vi "ArdnoTimedValves.vi"() -> ()   [LabVIEW 2018, in "Arduino.lvlib"]
uses:
  Backup LabVIEW Arduino Connection/LINX/Public/Peripherals/Digital/Digital Write N Chans.vi
  Arduino.lvlib
  Backup LabVIEW Arduino Connection/LINX/LVH-LINX.lvlib
panel:
  in  "Period [ms]":u32
  out "Error Out":errorcluster
  out "Device Name":string
  in  "error in (no error)":errorcluster
  in  "VISA resource name":refnum<visa-resource-name>
  in  "Manually controlled Valves":u8[](array[numeric])
  out "Open?":bool
  in  "Manual Open":bool
  in  "stop":bool
  # "ALWAYS TERMINATE THE\nPROGRAM WITH THIS STOP BUTTON!"
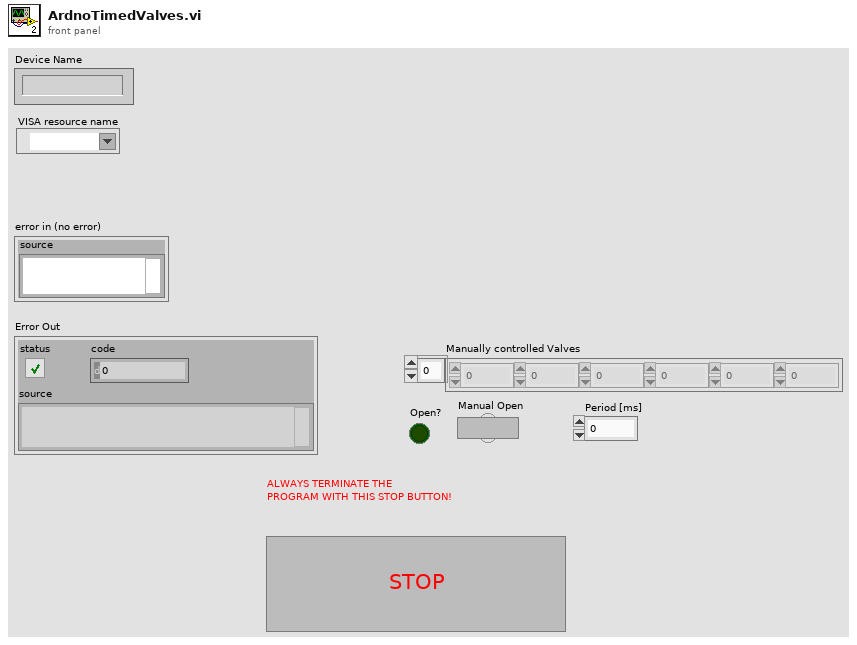
[diagram p1: front panel]
types:
  T1 = typedef "LVH-LINX.lvlib/LINX Ref.ctl" = cluster{"Platform":T2, "Interface":T3, "LINX Device Config":T4}
  T2 = typedef "LVH-LINX.lvlib/Platform.ctl" = enum16{"LINX", "myRIO"}
  T3 = typedef "LVH-LINX.lvlib/Interface.ctl" = enum16{"Serial", "TCP"}
  T4 = typedef "LVH-LINX.lvlib/Device.lvlib/LINX Device Config.ctl" = cluster{"Interface":T3, "COM Port":refnum<visa-resource-name>, "TCP Configuration":T5, "Device Family":T6, "Device ID":u8, "Device Name":string, "TCP Ref":refnum<k5>}
  T5 = typedef "LVH-LINX.lvlib/Device.lvlib/TCP Config.ctl" = cluster{"IP Address":string, "Port":u16}
  T6 = typedef "LVH-LINX.lvlib/Device Family.ctl" = enum8{"National Instruments", "Digilent", "Arduino"}
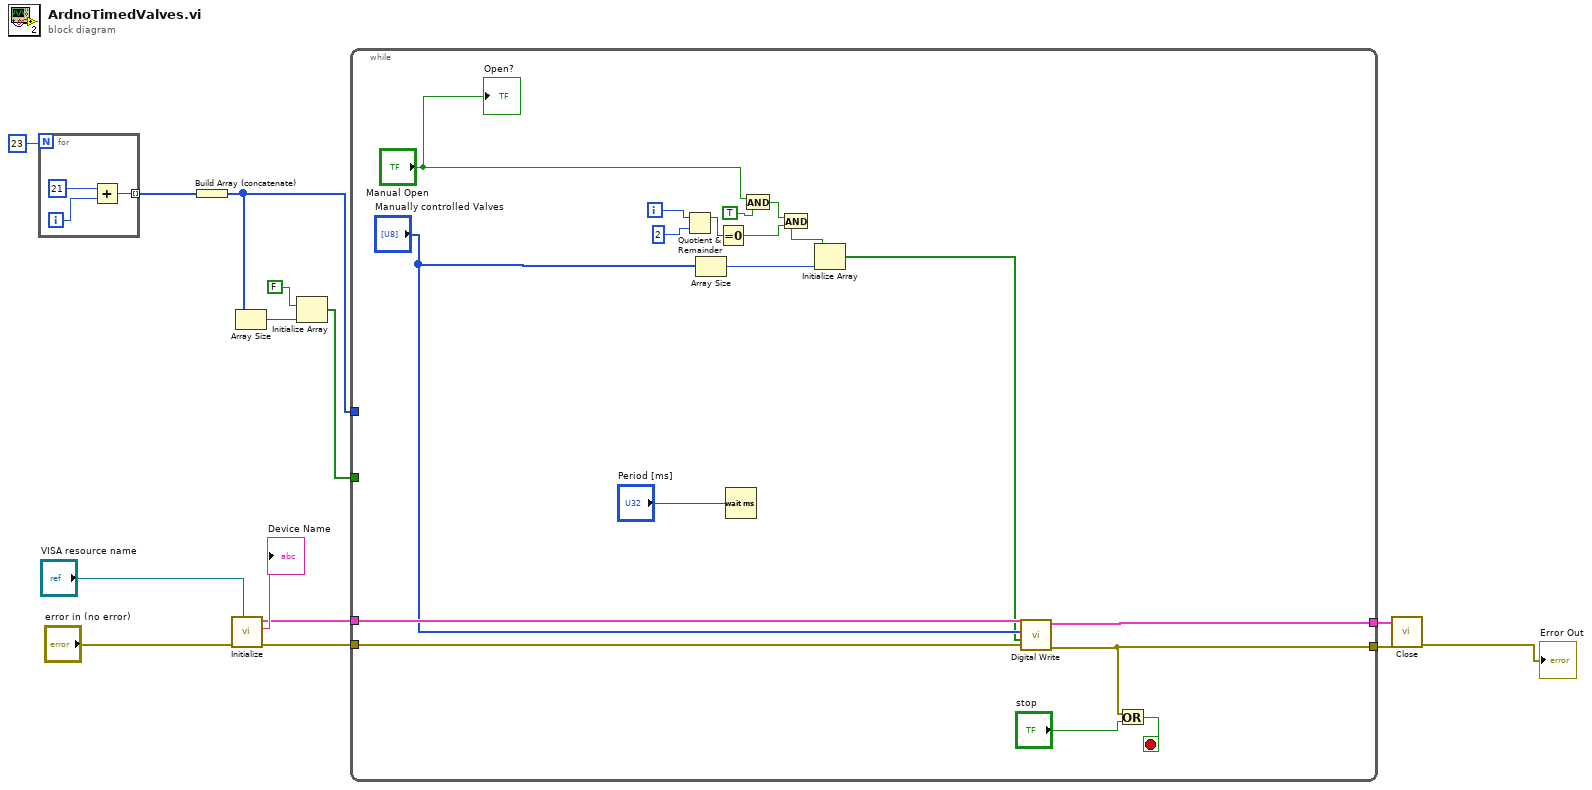
[diagram p0: block diagram]
diagram:
  n1 = for {
    N: 23 -> [_]
    tunnel: [w15] -> w5 mode=indexing
    i -> [w17]
    n2 = Add(x=21, y=w17) -> (x+y=w15:i32)
  }
  n3 = Build Array (concatenate)(w5) -> (w4:i32[])
  n4 = call "Initialize.vi"("Serial Port"="VISA resource name", "Error In"="error in (no error)") -> ("Error Out"=w7:errorcluster, "Device Name"=→"Device Name":string, "LINX Ref"=w8:T1)  [unwired: 7 in]
  n5 = Array Size(array=w4) -> (size(s)=w3:i32)
  n6 = Initialize Array(FALSE, w3) -> (w1:bool[])
  n7 = while {
    tunnel: w8 -> [w35]
    tunnel: [w34] -> w10
    tunnel: w7 -> [w33]
    tunnel: [w30] -> w9
    tunnel: w4 -> [_]
    tunnel: w1 -> [_]
    i -> [w20]
    stop <- w31 stop-if-true
    n8 = Quotient & Remainder(x=w20, y=2) -> (x-y*floor(x/y)=w25:i32)  [unwired: 1 out]
    n9 = Array Size(array="Manually controlled Valves") -> (size(s)=w23:i32)
    n10 = Equal To 0?(x=w25) -> (x = 0?=w28:bool)
    n11 = Wait (ms)(milliseconds to wait="Period [ms]") -> ()  [unwired: 1 out]
    n12 = And(x="Manual Open", y=TRUE) -> (x .and. y?=w29:bool)
    n13 = And(x=w29, y=w28) -> (x .and. y?=w27:bool)
    n14 = Initialize Array(w27, w23) -> (w19:bool[])
    n15 = call-poly "Digital Write.vi"("Error In"=w33, "Values"=w19, "DO Channels"="Manually controlled Valves", "LINX Resource"=w35) -> ("Error Out"=w30:errorcluster, "LINX Resource"=w34:T1)  [unwired: 6 in]
    n16 = Or(x=w30, y="stop") -> (x .or. y?=w31:bool)
    "Open?" <- "Manual Open"
  }
  n17 = call "Close.vi"("Error In"=w9, "LINX Resource"=w10) -> ("Error Out"=→"Error Out":errorcluster)  [unwired: 8 in, 1 out]
